vi "test_Multiple Local Array Type Cast Channel Command-Response Messages using Trigger.vi"(8 "error in (no error)":errorcluster, 11 "TestCase in":refnum<class "Instrument Addon Common System Tests.lvclass">) -> (0 "error out":errorcluster, 3 "TestCase out":refnum<class "Instrument Addon Common System Tests.lvclass">)   [LabVIEW 2020, in "Instrument Addon Common System Tests.lvclass"]
uses:
  Instrument Addon Common System Tests.lvclass
  C:/Program Files (x86)/National Instruments/LabVIEW 2020/vi.lib/NI/VeriStand Custom Device Testing Tools/VeriStandTestCase/VeriStandTestCase.lvclass
  <vilib>/NI VeriStand/Execution/Workspace/NI VeriStand - Set Multiple Channel Values.vi
  <vilib>/NI VeriStand/Execution/Workspace/NI VeriStand - Get Multiple Channel Values.vi
  <vilib>/addons/_JKI Toolkits/VI Tester/TestCase.llb/TestCase.lvclass
  <vilib>/NI VeriStand/Execution/Workspace/NI_VS Workspace ExecutionAPI.lvlib
  C:/Program Files (x86)/National Instruments/LabVIEW 2020/vi.lib/addons/_JKI Toolkits/VI Tester/TestCase.llb/TestCase.lvclass
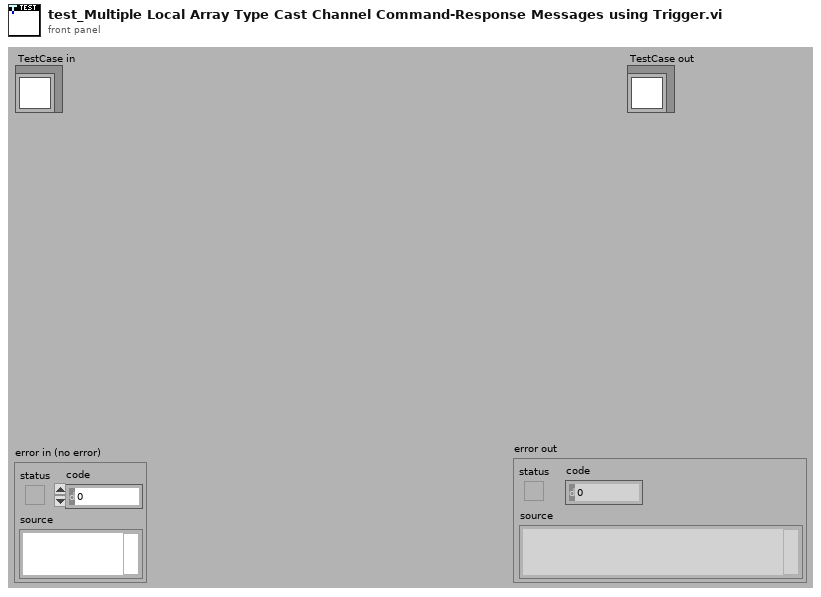
[diagram p1: front panel]
types:
  T1 = typedef "NI_VS Workspace ExecutionAPI.lvlib/WorkspaceAPI.ctl" = refnum<k24>
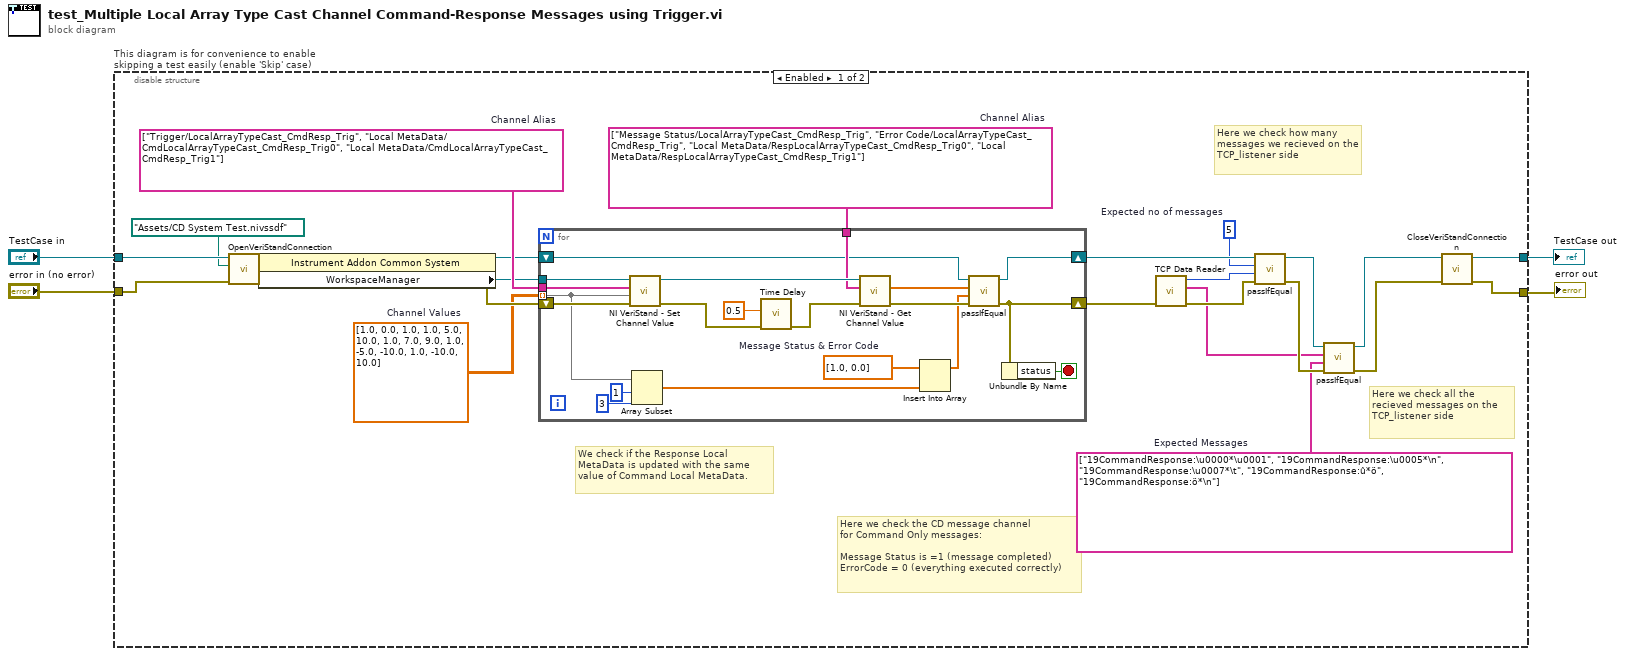
[diagram p0: block diagram]
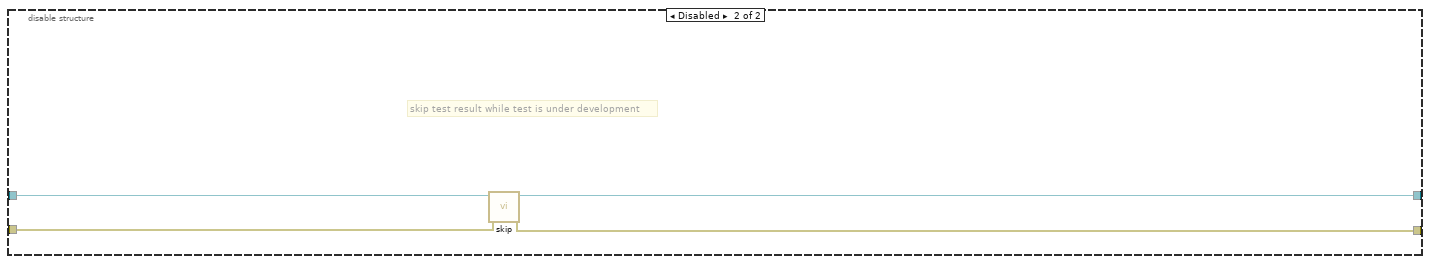
[diagram p2: hidden frame]
diagram:
  n1 = disable-structure "This diagram is for convenience to enable skipping a test easily (enable 'Skip' case)" shown="Enabled" {
    disable-tunnel: "TestCase in" -> [w26 w52]
    disable-tunnel: [w27 w50] -> w1
    disable-tunnel: [w28 w51] -> w3
    disable-tunnel: "error in (no error)" -> [w24 w49]
    frame Enabled {
      w5 = string[] ["19CommandResponse:\u0000*\u0001", "19CommandResponse:\u0005*\n", "19CommandResponse:\u0007*\t", "19CommandResponse:û*ö", "19CommandResponse:ö*\n"]  # Expected Messages
      w8 = 5  # Expected no of messages
      w17 = string[] ["Message Status/LocalArrayTypeCast_CmdResp_Trig", "Error Code/LocalArrayTypeCast_CmdResp_Trig", "Local MetaData/RespLocalArrayTypeCast_CmdResp_Trig0", "Local MetaData/RespLocalArrayTypeCast_CmdResp_Trig1"]  # Channel Alias
      w19 = dbl[][] [[1.0, 0.0, 1.0], [1.0, 5.0, 10.0], [1.0, 7.0, 9.0], [1.0, -5.0, -10.0], [1.0, -10.0, 10.0]]  # Channel Values
      w20 = string[] ["Trigger/LocalArrayTypeCast_CmdResp_Trig", "Local MetaData/CmdLocalArrayTypeCast_CmdResp_Trig0", "Local MetaData/CmdLocalArrayTypeCast_CmdResp_Trig1"]  # Channel Alias
      # "We check if the Response Local MetaData is updated with the same value of Command Local MetaData."
      # "Here we check how many messages we recieved on the TCP_listener side"
      # "Here we check all the recieved messages on the TCP_listener side"
      # "Here we check the CD message channel\nfor Command Only messages:\n\nMessage Status is =1 (message completed)\nErrorCode = 0 (everything executed correctly)"
      n2 = call-dynamic "OpenVeriStandConnection.vi"("error in (no error)"=w24, "System Definition File"=path "Assets/CD System Test.nivssdf", "VeriStand Test Case in"=w26) -> ("error out"=w23:errorcluster, "VeriStand Test Case out"=w25:refnum<class "Instrument Addon Common System Tests.lvclass">)  [unwired: 6 in, 1 out]
      n3 = property class="Instrument Addon Common System "(reference=w25, error in=w23) -> (reference out=w18:refnum<class "Instrument Addon Common System Tests.lvclass">, error out=w21:errorcluster, "WorkspaceManager"=w16:T1)
      n4 = for {
        tunnel: w16 -> [w48]
        tunnel: w20 -> [w46]
        tunnel: w19 -> [w33] mode=indexing
        shift-right: [w35] -> w7
        shift-left: w21 -> [w47]
        tunnel: w17 -> [w44]
        shift-right: [w39] -> w15
        shift-left: w18 -> [w40]
        stop <- w34 stop-if-true
        w36 = dbl[] [1.0, 0.0]  # Message Status & Error Code
        n5 = call-poly <vilib>:"NI VeriStand - Set Channel Value.vi"("error in (no error)"=w47, "Values"=w33, "Channels"=w46, "WorkspaceManager in"=w48) -> ("error out"=w42:errorcluster, "WorkspaceManager out"=w45:T1)  [unwired: 6 in]
        n6 = Array Subset(array=w33, index=1, length=3 ("index")) -> (w30:dbl[])
        n7 = call "Time Delay"("error in (no error)"=w42, "Delay Time (s)"=0.5) -> ("error out"=w41:errorcluster)  [unwired: 9 in]
        n8 = call-poly <vilib>:"NI VeriStand - Get Channel Value.vi"("error in (no error)"=w41, "Channels"=w44, "WorkspaceManager in"=w45) -> ("error out"=w38:errorcluster, "Values"=w37:dbl[])  [unwired: 6 in, 1 out]
        n9 = Insert Into Array(array=w36, new element=w30) -> (w32:dbl[])  [unwired: 1 in]
        n10 = call-dynamic "passIfEqual.vi"("error in (no error)"=w38, "y"=w32, "x"=w37, "TestCase in"=w40) -> ("error out"=w35:errorcluster, "TestCase out"=w39:refnum<class "Instrument Addon Common System Tests.lvclass">)  [unwired: 6 in]
        n11 = Unbundle By Name(w35) -> ("status"=w34:bool)
      }
      n12 = call "TCP Data Reader.vi"("error in (no error)"=w7) -> ("error out"=w13:errorcluster, "Recieved Messages"=w6:string[], "No of messages"=w9:i32)  [unwired: 8 in]
      n13 = call-dynamic "passIfEqual.vi"("error in (no error)"=w13, "y"=w9, "x"=w8, "TestCase in"=w15) -> ("error out"=w11:errorcluster, "TestCase out"=w14:refnum<class "Instrument Addon Common System Tests.lvclass">)  [unwired: 6 in]
      n14 = call-dynamic "passIfEqual.vi"("error in (no error)"=w11, "y"=w5, "x"=w6, "TestCase in"=w14) -> ("error out"=w10:errorcluster, "TestCase out"=w12:refnum<class "Instrument Addon Common System Tests.lvclass">)  [unwired: 6 in]
      n15 = call-dynamic "CloseVeriStandConnection.vi"("error in (no error)"=w10, "VeriStand Test Case in"=w12) -> ("error out"=w28:errorcluster, "VeriStand Test Case out"=w27:refnum<class "Instrument Addon Common System Tests.lvclass">)  [unwired: 8 in]
    }
    frame Disabled {
      # "skip test result while test is under development"
      n16 = call <vilib>:"skip.vi"("error in (no error)"=w49, "TestCase in"=w52) -> ("error out"=w51:errorcluster, "TestCase out"=w50:refnum<class "Instrument Addon Common System Tests.lvclass">)  [unwired: 8 in]
    }
  }
  "error out" <- w3
  "TestCase out" <- w1
